vi "aa_write_func.vi"(5 "Aardvark Handle":i32 min=0, 6 "No Stop? (False)":bool, 7 "Address (0x50)":u16=80 max=1023 format="%.0x", 8 "error in (no error)":errorcluster, 9 "Combined Format? (False)":bool, 10 "10-bit Addressing? (False)":bool, 11 "Data to Write":u8[](array[numeric]) format="%.0x") -> (0 "error out":errorcluster, 1 "Num Bytes Written":u16, 2 "Status":i32, 3 "dup Aardvark Handle":i32)   [LabVIEW 2014]
uses:
  aardvark-labview-x86_64-v5.15/aardvark-labview-x86_64-v5.15/aardvark.dll
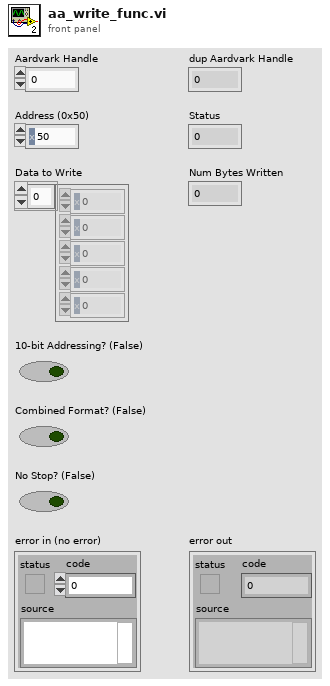
[diagram p1: front panel]
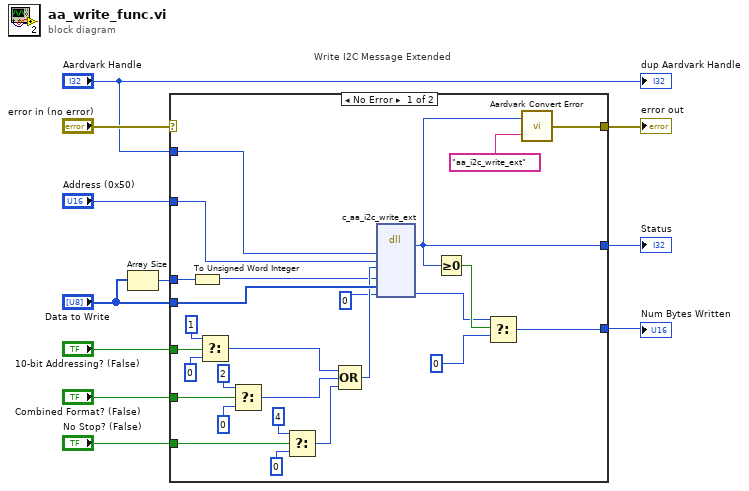
[diagram p0: block diagram]
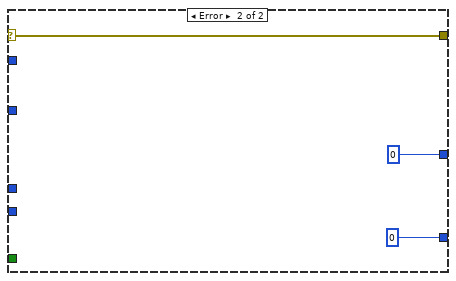
[diagram p2: hidden frame]
diagram:
  # "Write I2C Message Extended"
  n1 = Array Size(array="Data to Write") -> (size(s)=w8:i32)
  n2 = case shown="No Error" "error in (no error)" {
    selector: "error in (no error)" -> [_ w40]
    tunnel: [w36 w40] -> w1
    tunnel: "Aardvark Handle" -> [w35 _]
    tunnel: "Address (0x50)" -> [w34 _]
    tunnel: "10-bit Addressing? (False)" -> [w31 _]
    tunnel: "Combined Format? (False)" -> [w30 _]
    tunnel: "No Stop? (False)" -> [w29 _]
    tunnel: w8 -> [w16 _]
    tunnel: "Data to Write" -> [w18 _]
    tunnel: [w19 0] -> w10
    tunnel: [w13 0] -> w11
    frame No Error {
      n3 = To Unsigned Word Integer(number=w16) -> (unsigned 16bit integer=w12:u16)
      n4 = Select(t=1, s=w31, f=0) -> (s? t:f=w22:i32)
      n5 = Select(t=2, s=w30, f=0) -> (s? t:f=w21:i32)
      n6 = Select(t=4, s=w29, f=0) -> (s? t:f=w20:i32)
      n7 = Compound Arithmetic op=OR(w22, w21, w20) -> (w17:i32)
      n8 = dll-call lib="C:/Users/F114744/Desktop/aardvark-labview-x86_64-v5.15/aardvark-labview-x86_64-v5.15/aardvark.*" fn="c_aa_i2c_write_ext"("aardvark"=w35, "slave_addr"=w34, "flags"=w17, "num_bytes"=w12, "data_out"=w18, "num_written"=u16 0) -> (w13:i32, "num_written"=w14:u16)  [unwired: 8 in, 2 out]
      n9 = Greater Or Equal To 0?(x=w13) -> (x >= 0?=w33:bool)
      n10 = Select(t=w14, s=w33, f=u16 0) -> (s? t:f=w19:u16)
      n11 = call "Aardvark Convert Error.vi"("Source"="aa_i2c_write_ext", "Error Code"=w13) -> ("error out"=w36:errorcluster)
    }
    frame Error {
    }
  }
  "error out" <- w1
  "Num Bytes Written" <- w10
  "Status" <- w11
  "dup Aardvark Handle" <- "Aardvark Handle"
